vi "Init.vi"(6 "Post Meas?":bool, 7 "Prepend Result Name":bool, 8 "error in (no error)":errorcluster, 9 "DC Pins":string[](array[string]), 10 "Measurement Name":string, 11 "Standard":string) -> (0 "error out":errorcluster, 3 "DC_IDD out":refnum<class "DC_IDD.lvclass">)   [LabVIEW 2016, in "SeqAuto Evaluations.lvlib" / "DC_IDD.lvclass"]
uses:
  DC_IDD.lvclass
  C:/Sequence Automation/Plugins/SeqAuto IEvaluation.lvlibp/SeqAuto IEvaluation.lvclass
  DC_IDD.lvclass/DC_IDD.ctl
  Plugins/SeqAuto IEvaluation.lvlibp/Write Measurement Name.vi
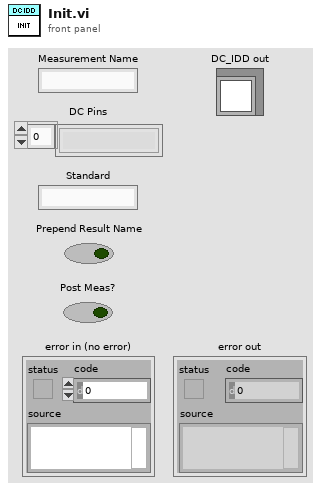
[diagram p1: front panel]
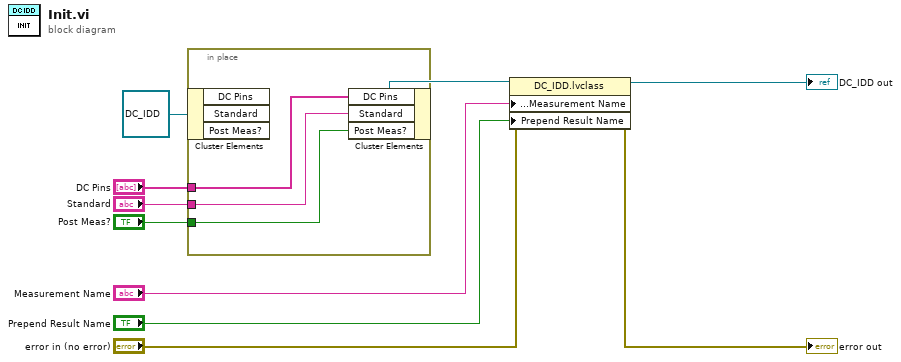
[diagram p0: block diagram]
diagram:
  n1 = in-place {
    in-place-border: "DC Pins" -> [w13]
    in-place-border: "Standard" -> [w12]
    in-place-border: "Post Meas?" -> [w11]
    n2 = in-place-cluster #1(refnum<class "DC_IDD.lvclass"> refnum ("DC_IDD in")) -> ()  [unwired: 3 out]
    n3 = in-place-cluster #1("DC Pins"=w13, "Standard"=w12, "Post Meas?"=w11) -> (w6:refnum<class "DC_IDD.lvclass">)
  }
  n4 = property class="DC_IDD.lvclass"(reference=w6, error in="error in (no error)", "Protected Methods:Measurement Name"="Measurement Name", "Prepend Result Name"="Prepend Result Name") -> (reference out=→"DC_IDD out":refnum<class "DC_IDD.lvclass">, error out=→"error out":errorcluster)
